vi "Read ColumnNameEqualsValueFormat.vi"(8 "error in (no error)":errorcluster, 11 "SqlMapper in":refnum<class "SqlMapper.lvclass">) -> (0 "error out":errorcluster, 2 "ColumnNameEqualsValueFormat":string="[%s] = @%s", 3 "SqlMapper out":refnum<class "SqlMapper.lvclass">)   [LabVIEW 2020, in "ORM.lvlib" / "SqlMapper.lvclass"]
uses:
  SqlMapper.lvclass
  DbConnection/DbConnection.lvclass
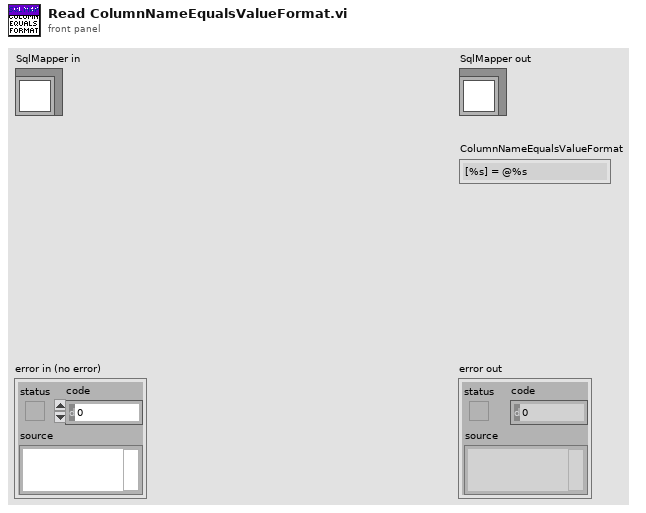
[diagram p1: front panel]
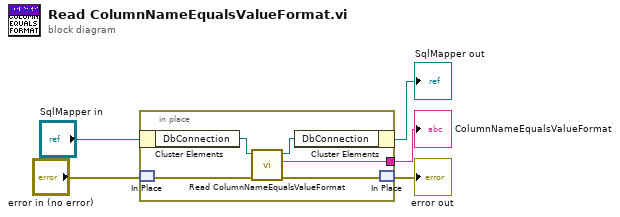
[diagram p0: block diagram]
diagram:
  n1 = in-place {
    in-place-border: [w8] -> w5
    n2 = in-place-cluster #1("SqlMapper in") -> ("DbConnection"=w10:refnum<class "DbConnection.lvclass">)
    n3 = in-place-match #2("error in (no error)") -> (w6:errorcluster)
    n4 = call "Read ColumnNameEqualsValueFormat.vi"("error in (no error)"=w6, "DbConnection in"=w10) -> ("error out"=w7:errorcluster, "ColumnNameEqualsValueFormat"=w8:string, "DbConnection out"=w9:refnum<class "DbConnection.lvclass">)  [unwired: 7 in]
    n5 = in-place-cluster #1("DbConnection"=w9) -> (→"SqlMapper out":refnum<class "SqlMapper.lvclass">)
    n6 = in-place-match #2(w7) -> (→"error out":errorcluster)
  }
  "ColumnNameEqualsValueFormat" <- w5
